vi "detect event type.vi"(6 "OldVal":string, 8 "NewVal":string) -> (0 "diff":string, 1 "#":i32, 2 "NewVal dup":string, 3 "event":T1=enum."no change")   [LabVIEW 2010, in "password.xctl"]
uses:
  password.xctl
  controls/Events.ctl
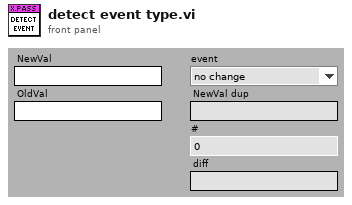
[diagram p1: front panel]
types:
  T1 = typedef "Events.ctl" = enum16{"first car", "add car", "remove car", "bad change", "no change"}
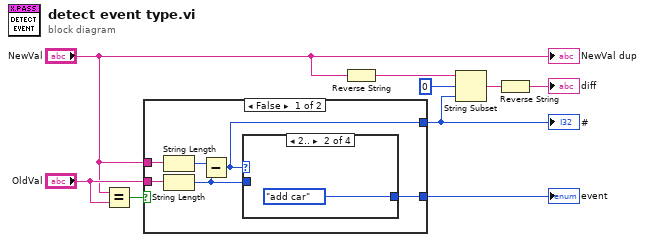
[diagram p0: block diagram]
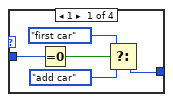
[diagram p2: hidden frame]
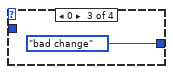
[diagram p3: hidden frame]
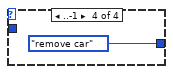
[diagram p4: hidden frame]
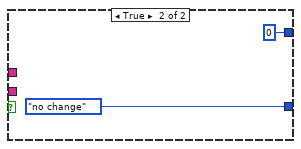
[diagram p5: hidden frame]
diagram:
  n1 = Equal?(x="NewVal", y="OldVal") -> (x = y?=w9:bool)
  n2 = case shown="False" w9 {
    tunnel: [w11 Events."no change"] -> w8
    tunnel: "NewVal" -> [w15 _]
    tunnel: "OldVal" -> [w14 _]
    tunnel: [w12 0] -> w2
    frame False {
      n3 = String Length(string=w15) -> (length=w13:i32)
      n4 = String Length(string=w14) -> (length=w10:i32)
      n5 = Subtract(x=w13, y=w10) -> (x-y=w12:i32)
      n6 = case shown="2.." w12 {
        tunnel: [w19 Events."add car" Events."bad change" Events."remove car"] -> w11
        tunnel: w10 -> [w18 _ _ _]
        frame 1 {
          n7 = Equal To 0?(x=w18) -> (x = 0?=w17:bool)
          n8 = Select(t=Events."first car", s=w17, f=Events."add car") -> (s? t:f=w19:T1)
        }
        frame 2.. {
        }
        frame 0 {
        }
        frame ..-1 {
        }
      }
    }
    frame True {
    }
  }
  "event" <- w8
  "#" <- w2
  n9 = Reverse String(1:"NewVal") -> (0:w5:string)
  n10 = String Subset(string=w5, offset (0)=0, length (rest)=w2) -> (substring=w3:string)
  n11 = Reverse String(1:w3) -> (0:→"diff":string)
  "NewVal dup" <- "NewVal"
